vi "DPT Estimate Completion Time.vi"(0 "IMC Weight":dbl, 5 "Completion Weight":dbl, 7 "Time Values":dbl[](array[numeric]), 9 "Weight Values":dbl[](array[numeric])) -> (4 "Completion Time Estimate":dbl, 6 "Prediction":dbl[](array[numeric]), 8 "Time Array":dbl[](array[numeric]))   [LabVIEW 2016]
uses:
  <vilib>/Analysis/NI_AALPro.lvlib
  <vilib>/gmath/NI_Gmath.lvlib
panel:
  in  "parameter bounds":T1={"amp min"=-inf, "amp max"=inf, "damping min"=-inf, "damping max"=inf, "offset min"=0.0, "offset max"=0.0}
  in  "method":u16(ring)=1 items=["Least Square", "Least Absolute Residual", "Bisquare"]
  out "residue":dbl
  out "damping":dbl
  out "amplitude":dbl
  out "Exponential Model Graph":dbl[][](graph)
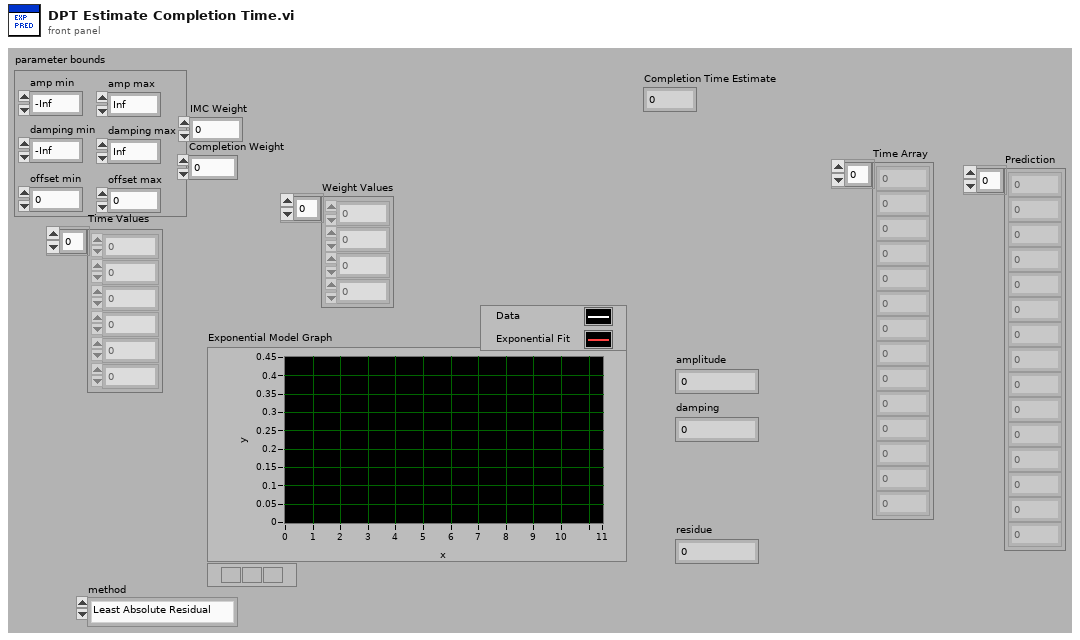
[diagram p1: front panel]
types:
  T1 = cluster{"amp min":dbl, "amp max":dbl, "damping min":dbl, "damping max":dbl, "offset min":dbl, "offset max":dbl}
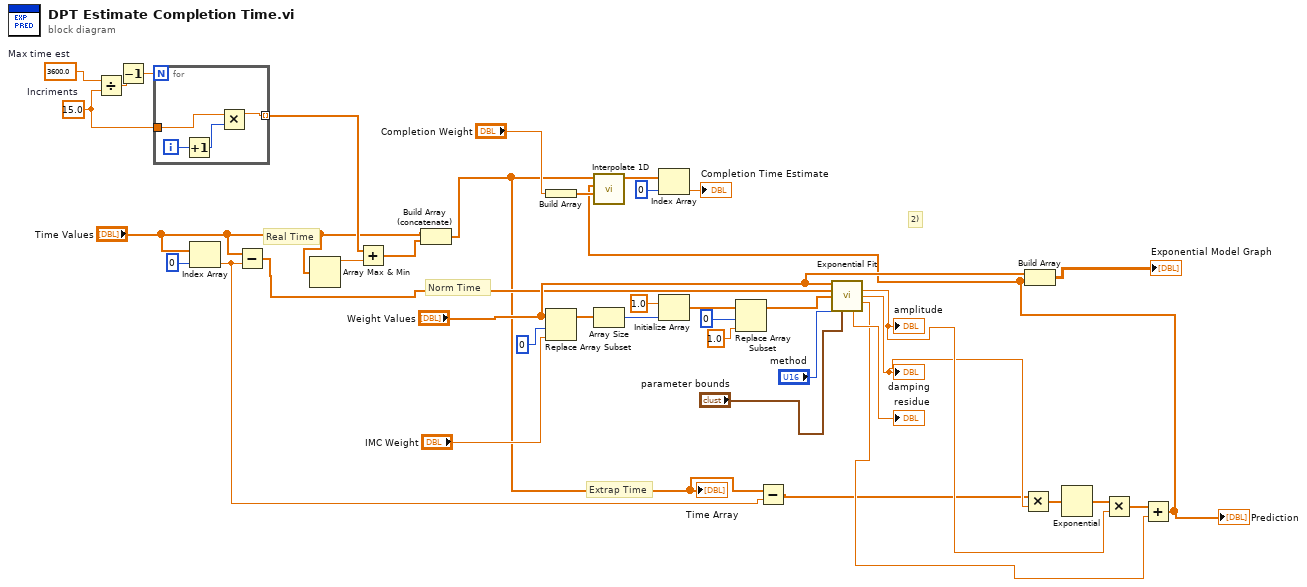
[diagram p0: block diagram]
diagram:
  w20 = 15.0  # Incriments
  w22 = 3600.0  # Max time est
  # "Extrap Time"
  # "Real Time"
  # "Norm Time"
  # "2)"
  n1 = Divide(x=w22, y=w20) -> (x/y=w21:dbl)
  n2 = Decrement(x=w21) -> (x-1=w5:dbl)
  n3 = for {
    N: w5 -> [_]
    tunnel: [w42] -> w18 mode=indexing
    tunnel: w20 -> [w41]
    i -> [w43]
    n4 = Increment(x=w43) -> (x+1=w40:i32)
    n5 = Multiply(x=w41, y=w40) -> (x*y=w42:dbl)
  }
  n6 = Index Array(array="Time Values", index=0) -> (element=w2:dbl)
  n7 = Subtract(x="Time Values", y=w2) -> (x-y=w14:dbl[])
  n8 = Array Max & Min(array="Time Values") -> (max value=w19:dbl)  [unwired: 3 out]
  n9 = Add(x=w18, y=w19) -> (x+y=w17:dbl[])
  n10 = Build Array (concatenate)("Time Values", w17) -> (w4:dbl[])
  "Time Array" <- w4
  n11 = Build Array("Completion Weight") -> (w26:dbl[])
  n12 = Replace Array Subset(array="Weight Values", new element="IMC Weight", index=0) -> (w30:dbl[])
  n13 = Array Size(array=w30) -> (size(s)=w37:i32)
  n14 = Initialize Array(1.0 ("element"), w37) -> (w35:dbl[])
  n15 = Replace Array Subset(array=w35, new element=1.0 ("new element/subarray"), index=0) -> (w32:dbl[])
  n16 = Subtract(x=w4, y=w2) -> (x-y=w3:dbl[])
  n17 = call <vilib>:"Exponential Fit.vi"("Y"="Weight Values", "X"=w14, "Weight"=w32, "method"="method", "parameter bounds"="parameter bounds") -> ("amplitude"=w10:dbl, "damping"=w9:dbl, "offset"=w8:dbl, "residue"=→"residue":dbl)  [unwired: 5 in, 2 out]
  "amplitude" <- w10
  "damping" <- w9
  n18 = Multiply(x=w3, y=w9) -> (x*y=w13:dbl[])
  n19 = Exponential(1:w13) -> (0:w12:dbl[])
  n20 = Multiply(x=w12, y=w10) -> (x*y=w11:dbl[])
  n21 = Add(x=w11, y=w8) -> (x+y=w7:dbl[])
  "Prediction" <- w7
  n22 = call <vilib>:"Interpolate 1D.vi"("xi"=w26, "X"=w7, "Y"=w4) -> ("yi"=w29:dbl[])  [unwired: 6 in, 2 out]
  n23 = Index Array(array=w29, index=0) -> (element=→"Completion Time Estimate":dbl)
  n24 = Build Array("Weight Values", w7) -> (→"Exponential Model Graph":dbl[][])
